vi "JoyPack.vi"(5 "Axes":dbl[](array[numeric]), 7 "Buttons":bool[](array[boolean])) -> (6 "JoyStick":T1)   [LabVIEW 2018]
uses:
  Typedefs/typedef_cluster_Joystick.ctl
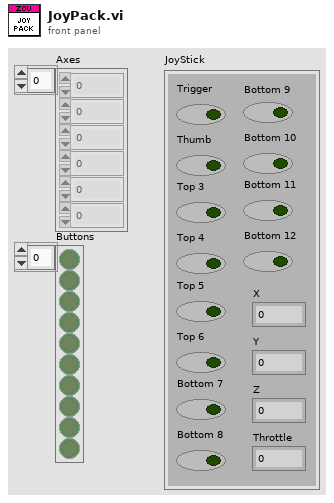
[diagram p1: front panel]
types:
  T1 = typedef "typedef_cluster_Joystick.ctl" = cluster{"X":dbl, "Y":dbl, "Z":dbl, "Throttle":dbl, "Trigger":bool, "Thumb":bool, "Top 3":bool, "Top 4":bool, "Top 5":bool, "Top 6":bool, "Bottom 7":bool, "Bottom 8":bool, "Bottom 9":bool, "Bottom 10":bool, "Bottom 11":bool, "Bottom 12":bool}
  T2 = cluster{"upper limit":dbl, "upper limit":dbl, "upper limit":dbl, "upper limit":dbl, bool, bool, bool, bool, bool, bool, bool, bool, bool, bool, bool, bool}
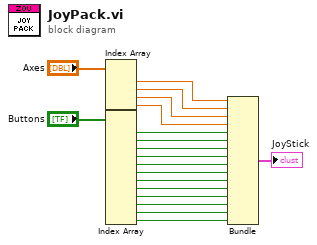
[diagram p0: block diagram]
diagram:
  n1 = Index Array(array="Axes") -> (element #1=w19:dbl, element #2=w17:dbl, element #3=w16:dbl, element #4=w15:dbl)  [unwired: 4 in]
  n2 = Index Array(array="Buttons") -> (element #1=w14:bool, element #2=w13:bool, element #3=w12:bool, element #4=w11:bool, element #5=w10:bool, element #6=w9:bool, element #7=w8:bool, element #8=w7:bool, element #9=w6:bool, element #10=w5:bool, element #11=w4:bool, element #12=w3:bool)  [unwired: 12 in]
  n3 = Bundle("upper limit"=w19, "upper limit"=w17, "upper limit"=w16, "upper limit"=w15, w14, w13, w12, w11, w10, w9, w8, w7, w6, w5, w4, w3) -> (→"JoyStick":T2)  [unwired: 1 in]
